vi "WPI_CameraDetermine Camera Type.vi"(8 "NT Connection":bool, 9 "Camera Name":string, 10 "iteration":i32) -> (1 "Camera Type":enum16{"None", "USB", "IP"}(ring), 2 "port":i32, 3 "address":string, 4 "cgi string":string, 5 "parameters":T1(array[cluster]))   [LabVIEW 2017]
uses:
  <vilib>/Rock Robotics/Network Tables/NT Read String Array.vi
  <vilib>/Rock Robotics/Network Tables/NT Read String.vi
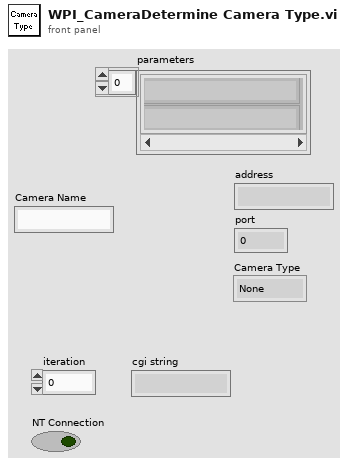
[diagram p1: front panel]
types:
  T1 = cluster{"token string":string, "token string 2":string}[]
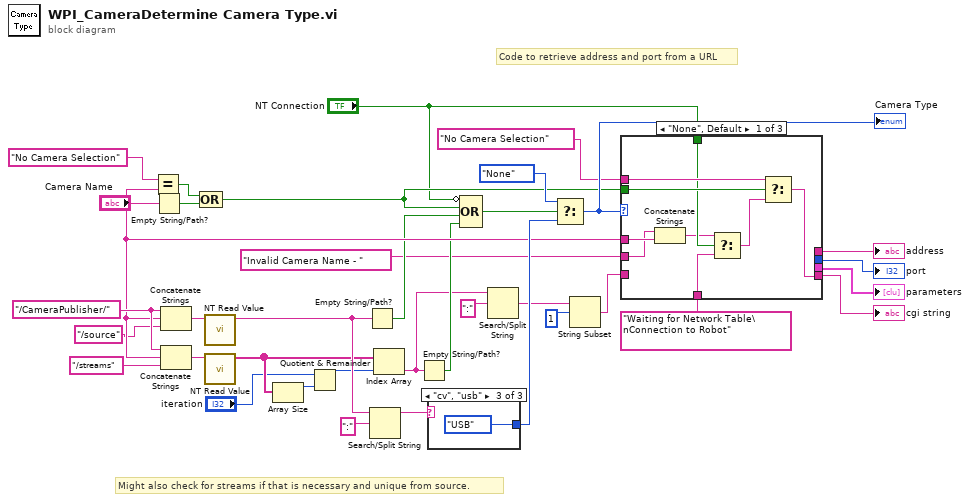
[diagram p0: block diagram]
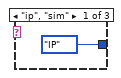
[diagram p2: hidden frame]
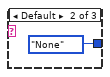
[diagram p3: hidden frame]
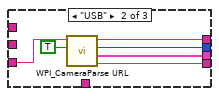
[diagram p4: hidden frame]
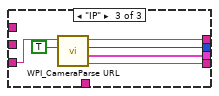
[diagram p5: hidden frame]
diagram:
  w30 = "/CameraPublisher/"
  # "Code to retrieve address and port from a URL"
  # "Might also check for streams if that is necessary and unique from source."
  n1 = Equal?(x="No Camera Selection", y="Camera Name") -> (x = y?=w8:bool)
  n2 = Empty String/Path?(string/path="Camera Name") -> (empty?=w7:bool)
  n3 = Concatenate Strings(w30, "Camera Name", "/source") -> (w32:string)
  n4 = Concatenate Strings(w30, "Camera Name", "/streams") -> (w28:string)
  n5 = Compound Arithmetic op=OR(w8, w7) -> (w6:bool)
  n6 = call-poly <vilib>:"NT Read Value.vi"("Name"=w32) -> ("String"=w18:string)  [unwired: 9 in, 1 out]
  n7 = call-poly <vilib>:"NT Read Value.vi"("Name"=w28) -> ("String Array"=w15:string[])  [unwired: 9 in, 1 out]
  n8 = Array Size(array=w15) -> (size(s)=w14:i32)
  n9 = Quotient & Remainder(x="iteration", y=w14) -> (x-y*floor(x/y)=w16:i32)  [unwired: 1 out]
  n10 = Empty String/Path?(string/path=w18) -> (empty?=w12:bool)
  n11 = Search/Split String(string=w18, search string/char (-)=":" ("format string")) -> (substring before match=w17:string)  [unwired: 1 in, 2 out]
  n12 = Index Array(array=w15, index=w16) -> (element=w24:string)
  n13 = Empty String/Path?(string/path=w24) -> (empty?=w27:bool)
  n14 = case shown="\"cv\", \"usb\"" w17 {
    tunnel: [enum16{"None", "USB", "IP"}."IP" ("Enum") enum16{"None", "USB", "IP"}."None" ("Enum") enum16{"None", "USB", "IP"}."USB" ("Enum")] -> w31
    frame "ip", "sim" {
    }
    frame Default {
    }
    frame "cv", "usb" {
    }
  }
  n15 = Compound Arithmetic op=OR(invert "NT Connection", w6, w12, w27) -> (w33:bool)
  n16 = Search/Split String(string=w24, search string/char (-)=":" ("format string")) -> (match + rest of string=w22:string)  [unwired: 1 in, 2 out]
  n17 = Select(t=enum16{"None", "USB", "IP"}."None" ("Enum"), s=w33, f=w31) -> (s? t:f=w35:enum16{"None", "USB", "IP"})
  "Camera Type" <- w35
  n18 = String Subset(string=w22, offset (0)=1) -> (substring=w20:string)  [unwired: 1 in]
  n19 = case shown="\"None\", Default" w35 {
    tunnel: [_ w52 w58] -> w3
    tunnel: "Camera Name" -> [w48 _ _]
    tunnel: w20 -> [_ w53 w59]
    tunnel: "No Camera Selection" -> [w45 _ _]
    tunnel: [_ w51 w57] -> w10
    tunnel: [_ w50 w56] -> w9
    tunnel: [w40 w49 w55] -> w2
    tunnel: w6 -> [w47 _ _]
    tunnel: "Invalid Camera Name - " -> [w46 _ _]
    tunnel: "NT Connection" -> [w44 _ _]
    tunnel: "Waiting for Network Table\nConnection to Robot" -> [w43 _ _]
    frame "None", Default {
      n20 = Concatenate Strings(w46, w48) -> (w42:string)
      n21 = Select(t=w42, s=w44, f=w43) -> (s? t:f=w41:string)
      n22 = Select(t=w45, s=w47, f=w41) -> (s? t:f=w40:string)
    }
    frame "USB" {
      n23 = call <vilib>:"WPI_CameraParse URL.vi"("Full"=TRUE, "URL"=w53) -> ("cgi string"=w49:string, "parameters"=w50:T1, "port"=w51:i32, "address"=w52:string)  [unwired: 6 in]
    }
    frame "IP" {
      n24 = call <vilib>:"WPI_CameraParse URL.vi"("Full"=TRUE, "URL"=w59) -> ("cgi string"=w55:string, "parameters"=w56:T1, "port"=w57:i32, "address"=w58:string)  [unwired: 6 in]
    }
  }
  "address" <- w3
  "port" <- w10
  "cgi string" <- w2
  "parameters" <- w9
